vi "VISP Snippet Read.vi"(8 "error in (no error)":errorcluster, 10 "VI Path (*.vi)":path, 11 "VI Snippet Path (*.png)":path) -> (0 "error out":errorcluster, 2 "dup VI Path":path, 3 "Image Data out":T1)   [LabVIEW 2019, in "VI Snippet.lvlib"]
doc: "Returns the <b>VI Snippet Path (*.png)</b> image and saves the embedded VI to the <b>VI Path (*.vi)</b> specified (from the \"niVI\" PNG chunk).\n\n<b>Errors:</b>\n1059: \"Unsupported file type\" if the \"niVI\" PNG chunk is not found.\n1065: \"Empty VI path\" if the <b>VI Path (*.vi)</b> is empty.\n\nCreated by: Ryan Pacini"
uses:
  VI Snippet.lvlib
  <vilib>/picture/picture.llb/imagedata.ctl
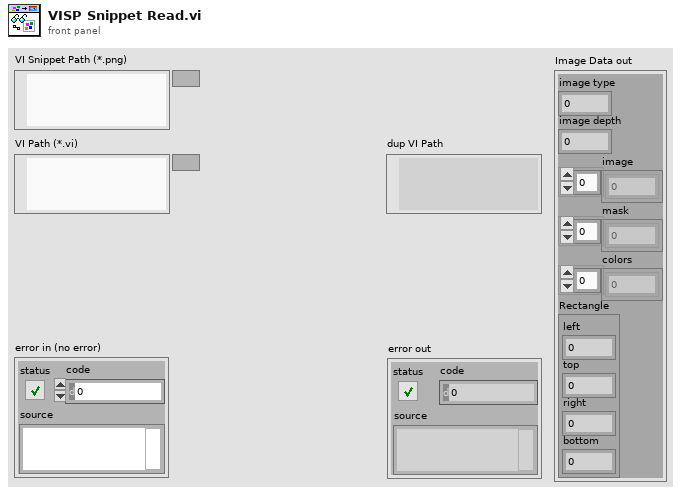
[diagram p1: front panel]
types:
  T1 = typedef "imagedata.ctl" = cluster{"image type":i32, "image depth":i32, "image":u8[], "mask":u8[], "colors":u32[], "Rectangle":cluster{"left":i16, "top":i16, "right":i16, "bottom":i16}}
  T2 = typedef "VI Snippet.lvlib/VISP PNG Chunk.ctl" = cluster{"Length":i32, "Type":string, "Data":string, "CRC":u32}
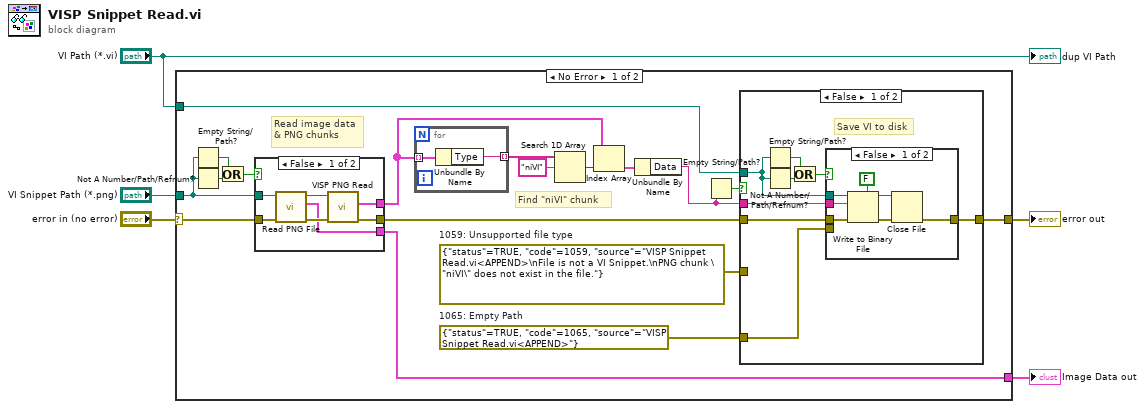
[diagram p0: block diagram]
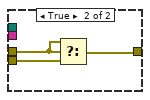
[diagram p3: hidden frame]
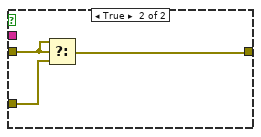
[diagram p4: hidden frame]
diagram:
  n1 = case shown="No Error" "error in (no error)" {
    selector: "error in (no error)" -> [w23 w55]
    tunnel: "VI Snippet Path (*.png)" -> [w10 _]
    tunnel: [w11 _] -> w3
    tunnel: [w16 w55] -> w2
    tunnel: "VI Path (*.vi)" -> [w15 _]
    frame No Error {
      w6 = errorcluster {"status"=TRUE, "code"=1065, "source"="VISP Snippet Read.vi<APPEND>"}  # 1065: Empty Path
      w12 = errorcluster {"status"=TRUE, "code"=1059, "source"="VISP Snippet Read.vi<APPEND>\nFile is not a VI Snippet.\nPNG chunk \"niVI\" does not exist in the file."}  # 1059: Unsupported file type
      # "Read image data\n& PNG chunks"
      # "Find \"niVI\" chunk"
      n2 = Empty String/Path?(string/path=w10) -> (empty?=w9:bool)
      n3 = Not A Number/Path/Refnum?(number/path/refnum=w10) -> (NaN/Path/Refnum?=w8:bool)
      n4 = Or(x=w9, y=w8) -> (x .or. y?=w7:bool)
      n5 = case shown="False" w7 {
        tunnel: w23 -> [w30 w31]
        tunnel: w10 -> [w29 _]
        tunnel: [w26 w31] -> w18
        tunnel: [w25 _] -> w13
        tunnel: [w24 _] -> w11
        frame False {
          n6 = call <vilib>:"Read PNG File.vi"("error in (no error)"=w30, "path to PNG file"=w29) -> ("error out"=w27:errorcluster, "image data"=w24:T1, "path"=w28:path)  [unwired: 7 in]
          n7 = call "VISP PNG Read.vi"("error in (no error)"=w27, "Image Path (*.png)"=w28) -> ("error out"=w26:errorcluster, "Chunks"=w25:T2[])  [unwired: 7 in, 1 out]
        }
        frame True {
        }
      }
      n8 = for {
        tunnel: w13 -> [w33] mode=indexing
        tunnel: [w32] -> w22 mode=indexing
        n9 = Unbundle By Name(w33) -> ("Type"=w32:string)
      }
      n10 = Search 1D Array(1D array=w22, element="niVI" ("Type")) -> (index of element=w20:i32)  [unwired: 1 in]
      n11 = Index Array(array=w13, index=w20) -> (element=w19:T2)
      n12 = Unbundle By Name(w19) -> ("Data"=w17:string)
      n13 = Empty String/Path?(string/path=w17) -> (empty?=w14:bool)
      n14 = case shown="False" w14 {
        tunnel: w18 -> [w41 w52]
        tunnel: w17 -> [w40 _]
        tunnel: [w39 w53] -> w16
        tunnel: w15 -> [w36 _]
        tunnel: w12 -> [_ w54]
        tunnel: w6 -> [w34 _]
        frame False {
          # "Save VI to disk"
          n15 = Empty String/Path?(string/path=w36) -> (empty?=w38:bool)
          n16 = Not A Number/Path/Refnum?(number/path/refnum=w36) -> (NaN/Path/Refnum?=w37:bool)
          n17 = Or(x=w38, y=w37) -> (x .or. y?=w35:bool)
          n18 = case shown="False" w35 {
            tunnel: w41 -> [w45 w51]
            tunnel: w40 -> [w44 _]
            tunnel: [w43 w49] -> w39
            tunnel: w36 -> [w42 _]
            tunnel: w34 -> [_ w50]
            frame False {
              n19 = Write to Binary File(file (use dialog)=w42, data=w44, error in=w45, 5:FALSE ("prepend array or string size? (T)")) -> (refnum out=w47:refnum<file>, error out=w48:errorcluster)  [unwired: 2 in, 1 out]
              n20 = Close File(refnum=w47, error in=w48) -> (error out=w43:errorcluster)  [unwired: 1 out]
            }
            frame True {
              n21 = Select(t=w51, s=w51, f=w50) -> (s? t:f=w49:errorcluster)
            }
          }
        }
        frame True {
          n22 = Select(t=w52, s=w52, f=w54) -> (s? t:f=w53:errorcluster)
        }
      }
    }
    frame Error {
    }
  }
  "error out" <- w2
  "Image Data out" <- w3
  "dup VI Path" <- "VI Path (*.vi)"
